vi "find index of the image name.vi"(8 "error in (no error)":errorcluster, 11 "Channel in":refnum<class "Channel.lvclass">) -> (0 "error out":errorcluster, 3 "Channel out":refnum<class "Channel.lvclass">)   [LabVIEW 2018, in "Channel.lvclass"]
doc: "Find the index of the lastest image in the current directory"
uses:
  Channel.lvclass
  Channel.lvclass/Channel.ctl
  Simulated_CCD_Camera/Simulated Camera.lvclass
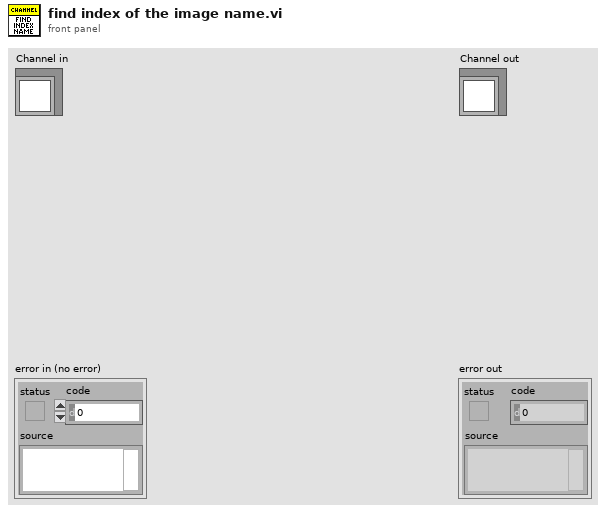
[diagram p1: front panel]
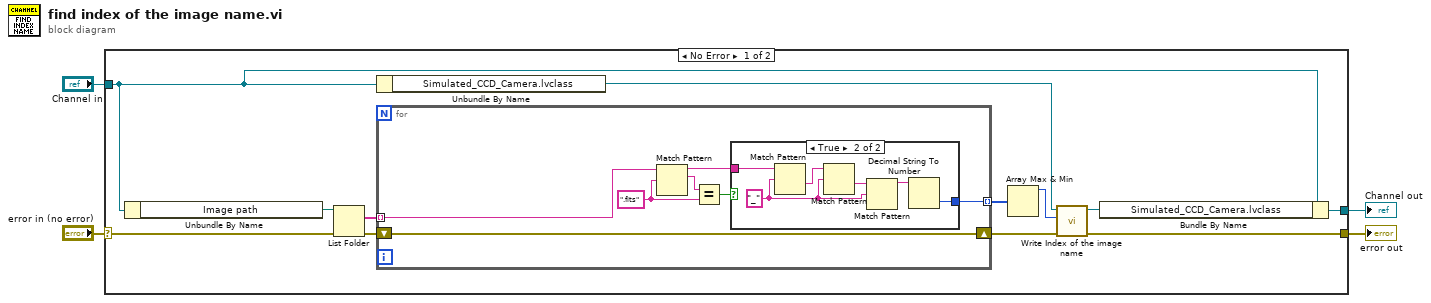
[diagram p0: block diagram]
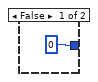
[diagram p2: hidden frame]
diagram:
  n1 = case shown="No Error" "error in (no error)" {
    selector: "error in (no error)" -> [w16 w32]
    tunnel: [w9 w32] -> w3
    tunnel: [w13 w31] -> w1
    tunnel: "Channel in" -> [w12 w31]
    frame No Error {
      n2 = Unbundle By Name(w12) -> ("Image path"=w5:path)
      n3 = List Folder(path=w5, error in=w16) -> (filenames=w14:string[], error out=w15:errorcluster)  [unwired: 2 in, 2 out]
      n4 = Unbundle By Name(w12) -> ("Simulated_CCD_Camera.lvclass"=w11:refnum<class "Simulated Camera.lvclass">)
      n5 = for {
        shift-right: [w23] -> w8
        shift-left: w15 -> [w23]
        tunnel: w14 -> [w20] mode=indexing
        tunnel: [w21] -> w7 mode=indexing
        w18 = ".fits" ("regular expression")
        n6 = Match Pattern(string=w20, regular expression=w18) -> (before substring=w22:string, match substring=w19:string)  [unwired: 1 in, 2 out]
        n7 = Equal?(x=w19, y=w18) -> (x = y?=w17:bool)
        n8 = case shown="True" w17 {
          tunnel: w22 -> [_ w29]
          tunnel: [0 w30] -> w21
          frame False {
          }
          frame True {
            w26 = "_" ("regular expression")
            n9 = Match Pattern(string=w29, regular expression=w26) -> (after substring=w28:string)  [unwired: 1 in, 3 out]
            n10 = Match Pattern(string=w28, regular expression=w26) -> (after substring=w27:string)  [unwired: 1 in, 3 out]
            n11 = Match Pattern(string=w27, regular expression=w26) -> (before substring=w25:string)  [unwired: 1 in, 3 out]
            n12 = Decimal String To Number(string=w25) -> (number=w30:i32)  [unwired: 2 in, 1 out]
          }
        }
      }
      n13 = Array Max & Min(array=w7) -> (max value=w6:i32)  [unwired: 3 out]
      n14 = call-dynamic "Write Index of the image name.vi"("error in (no error)"=w8, "Index of the image name"=w6, "Simulated_CCD_Camera in"=w11) -> ("error out"=w9:errorcluster, "Simulated_CCD_Camera out"=w10:refnum<class "Simulated Camera.lvclass">)  [unwired: 7 in]
      n15 = Bundle By Name(cluster=w12, "Simulated_CCD_Camera.lvclass"=w10) -> (w13:refnum<class "Channel.lvclass">)
    }
    frame Error {
    }
  }
  "error out" <- w3
  "Channel out" <- w1
